vi "SciScan RESONANT.vi"() -> ()   [LabVIEW 2017]
doc: "SciScan 1.1f2 160418"
uses:
  Custom Controls/Ch selector.ctl
  Custom Controls/MAIN Image panel reso tab Control type def.ctl
  Custom Controls/scan mode main settings tab.ctl
  Custom Controls/advanced settings inner tab CTL.ctl
  Custom Controls/Laser power 1 dial.ctl
  Custom Controls/Histogram tab reso.ctl
  Custom Controls/file format type def.ctl
  Custom Controls/display palette control.ctl
  Custom Controls/PositionSaveMod.ctl
  Custom Controls/pixel resolution resonant enum.ctl
  Custom Controls/experiment type.ctl
  HFG/Custom Controls and Typedefs/HFG Commands.ctl
  CommonResource VIs/Timing/Timer Commands.ctl
  HFG/SubVIs/Broken Chain FGV Command.ctl
  Plugins/Macro Module/Macro Rule/subVIs/MacroRules_FGV_Commands.ctl
  Plugins/Macro Module/Macro Rule/subVIs/MacroErrorsFGV_Commands.ctl
  <vilib>/event_ctls.llb/lveventtype.ctl
  INI/settingsIO/Settings IO_Commands.ctl
  Plugins/Macro Module/MacroGUI Module/Custom Controls and Typedefs/GFG Variable for IO.ctl
  <vilib>/Utility/miscctls.llb/LVMinMaxIncTypeDef.ctl
  <vilib>/Utility/miscctls.llb/LVOutOfRangeActionTypeDef.ctl
  <vilib>/DAQmx/write.llb/DAQmx Write (Analog DBL 1Chan 1Samp).vi
  GFG/GFGfpRefGet.vi
  <vilib>/DAQmx/miscellaneous.llb/DAQmx Fill In Error Info.vi
  GFG/GFGnumericGet.vi
  GFG/GFGpathGet.vi
  GFG/GFGstringGet.vi
  GFG/GFG library.lvlib
panel:
  in  "MAIN UI responsive? (F)":bool
  in  "shutterlock":bool caption="LOCK"
  in  "custom step z":bool
  in  "custom step xy":bool
  in  "no of grid lines":dbl(slide) min=0.0 step=1.0 scale=0.0..20.0
  out "grid size":string caption="GRID"
  in  "save prot":bool
  in  "piezo.active":bool
  in  "lasersync.enable":bool
  in  "resonant.correction.enable":bool
  in  "PositionSaveButton":T1
  in  "reset zoom":bool
  in  "bool.stage.speed":bool=TRUE
  in  "x.voltage":dbl=0.9999999999999999 min=0.0 max=5.5 step=0.1
  in  "y.voltage":dbl=1.0 min=0.0 max=5.5 step=0.1
  in  "y.volt.offset":dbl=-0.2 step=0.1
  in  "x.volt.offset":dbl=-0.2 step=0.1
  in  "shutter":bool
  in  "x.pixels":i32=256 min=2 max=2048 step=2
  in  "clear prot":bool
  in  "timestamp.prot":bool
  in  "protocol.notes":string caption="notebook"
  in  "Open All\nSettings":bool=TRUE
  in  "step.size.z":u16(ring)=1 items=["    1"=1, "    2"=2, "    5"=5, "  10"=10, "  20"=20, "100"=100]
  in  "Stage Stop":bool
  out "frame count":dbl(slide) scale=0.0..100.0
  in  "scan mode main settings":T2
  in  "pixel resolution":T3=enum."512 x 512"
  in  "autocorrect.startdelay":bool
  in  "x.correction":dbl(slide)=-27.0 min=-200.0 max=200.0 step=1.0 scale=-200.0..200.0 scale format="%#_3g"
  in  "ZOOM":dbl(slide)=1.0 min=1.0 max=20.1 step=0.125 scale=1.0..20.0
  in  "Start.Delay":dbl(slide)=1.0 min=1.0 max=2500.0 step=1.0 scale=1.0..2500.0 scale format="%#_3f"
  in  "no. of frames to acquire":i32=10000 min=4 max=1000000 step=4
  out "x.fov":dbl caption="Field of view    x" format="%#_3p"
  out "y.fov":dbl caption="y" format="%#_3p"
  out "frames.p.sec":dbl caption="frames/s" format="%#.2g"
  in  "invert.ch.4":bool
  in  "save.ch.4":bool caption="ch 4"
  in  "invert.ch.3":bool
  in  "save.ch.3":bool caption="ch 3"
  in  "invert.ch.2":bool
  in  "save.ch.2":bool caption="ch 2"
  in  "invert.ch.1":bool
  in  "save.ch.1":bool caption="ch 1"
  in  "experiment name":string
  in  "root.path":path=path "d:/"
  in  "file format":T4
  in  "experiment type":T5="XYT"
  in  "Objective":u16(ring) items=["Olympus 10x", "Olympus 60x", "Nikon 16x", "Olympus 25x"]
  out "stack.duration":i32=10 caption="stack.duration (sec)" min=0 max=2147483646 step=2
  in  "add":bool
  in  "clear all":bool
  in  "clear last":bool
  in  "move to z.stack.\nstart plane":bool
  in  "start z.stack":bool
  in  "frames.per.plane":i32=10000 min=4 max=1000000 step=4
  in  "z.spacing":dbl=1.0 caption="z.spacing (um)" min=0.1 step=0.1
  out "no of planes":i32=10 min=0 max=2147483646 step=2
  in  "piezo.mode":bool
  out "volume rate (in Hz)":dbl=1.0 min=0.0 max=5.5 step=0.1 format="%#.2g"
  in  "frames.per.z.cycle":dbl=4.0 min=4.0 step=2.0
  in  "no.of.cycles.to.scan":dbl=2.0 caption="no.of.volumes" min=1.0 step=1.0
  in  "piezo.offset.compensation.seconds":dbl caption="no.of.volumes"
  in  "Z UP":bool
  in  "Z DOWN":bool
  out "String 7":string
  in  "step.size.xy":u16(ring)=1 items=["   1"=1, "   2"=2, "   5"=5, "  10"=10, "  20"=20, "  50"=50, "100"=100]
  in  "Y UP":bool
  in  "X LEFT":bool
  in  "Y DOWN":bool
  in  "X RIGHT":bool
  out "String 6":string
  in  "setY":dbl caption="Z-Stepper" format="%#.1f"
  in  "setX":dbl caption="Z-Stepper" format="%#.1f"
  in  "setZ":dbl caption="set" format="%#.1f"
  out "String 4":string
  out "posZ":dbl caption="actual" format="%#.1f"
  out "posX":dbl caption="Z-Stepper" format="%#.1f"
  out "posY":dbl caption="Z-Stepper" format="%#.1f"
  out "String 3":string
  in  "QUIT":bool
  in  "Record":bool
  in  "FOCUS":bool
  in  "MAIN Image panels reso":T6
  out "Channel 1 large":T7(plugin-control)
  out "Channel 2 large":T7(plugin-control)
  out "Channel 3 large":T7(plugin-control)
  out "Channel 4 large":T7(plugin-control)
  out "Channel 5 large":T7(plugin-control)
  out "Channel 1 small":T7(plugin-control)
  out "Channel 2 small":T7(plugin-control)
  out "Channel 4 small":T7(plugin-control)
  out "Channel 3 small":T7(plugin-control)
  in  "Blue Channel (Overlay)":T8 caption="B"
  in  "Green Channel (Overlay)":T8=enum."Ch 1" caption="G"
  in  "Red Channel (Overlay)":T8=enum."Ch 2" caption="R"
  out "RGB overlay":T7(plugin-control)
  out "ROI chart":sgl[][](graph)=[[54.570076, 54.556858]]
  in  "ROI channel":T8=enum."Ch 1" caption="Channel"
  out "ROI Image display":T7(plugin-control)
  in  "confirm line":bool
  in  "channel arb line scan":T8 caption="Channel"
  out "arb line scan display":T7(plugin-control)
  in  "Cancel":bool
  in  "hist/ref slider tab":enum32{" "}(tab)
  in  "display every n-th frame":i8=4 min=2 step=1
  in  "PIN Button hist/ref slider tab":bool=TRUE
  in  "Histograms tab reso":T9
  in  "auto scale\n      CH 1":bool=TRUE caption="auto scale 2"
  in  "Min Max Channel 1":cluster{dbl, dbl}(slide)={0.0, 65535.0} scale=0.0..65535.0 scale format="%#_5g"
  out "Histogram 1":T10(graph)
  out "String 12":string
  in  "auto scale\n      CH 4":bool=TRUE caption="auto scale 2"
  in  "Min Max Channel 4":cluster{dbl, dbl}(slide)={0.0, 65535.0} scale=0.0..65535.0 scale format="%#_5g"
  out "Histogram 4":T10(graph)
  out "String 15":string
  in  "auto scale\n      CH 5":bool=TRUE caption="auto scale 2"
  in  "Min Max Channel 5":cluster{dbl, dbl}(slide) scale=-100.0..2047.0 scale format="%#_4g"
  out "Histogram 5":T10(graph)
  out "String 16":string
  in  "auto scale\n      CH 3":bool=TRUE caption="auto scale 2"
  in  "Min Max Channel 3":cluster{dbl, dbl}(slide)={0.0, 65535.0} scale=0.0..65535.0 scale format="%#.1f"
  out "Histogram 3":T10(graph)
  out "String 14":string
  in  "auto scale\n      CH 2":bool=TRUE caption="auto scale 2"
  in  "Min Max Channel 2":cluster{dbl, dbl}(slide)={0.0, 65535.0} scale=0.0..65535.0 scale format="%#.0f"
  out "Histogram 2":T10(graph)
  out "String 13":string
  in  "avg type":u16(ring) items=["none", "group avg", "moving avg"]
  in  "avg of":i8=10 min=2 step=1
  in  "display palette":T11
  in  "large histogram":bool caption="Pop-Out"
  in  "laser power slider tab":enum32{""}(tab)
  in  "enable set power max":bool
  in  "set power max":bool
  in  "Laser Power":T12 min=0.0 max=100.0 step=0.5 scale=0.0..100.0 scale format="%3d"
  in  "PIN Button laser power slider tab":bool=TRUE
  in  "blanking\npercentage":i32=90 min=0 max=90 step=1
  in  "PMT slider tab":enum32{""}(tab)
  in  "PMT 2":u16(slide) max=1000 scale=0.0..1000.0
  in  "PMT 1":u16(slide) max=1250 scale=0.0..1000.0
  out "String 5":string
  in  "PMT 4":u16(slide) max=1000 scale=0.0..1000.0
  in  "PMT 3":u16(slide) max=1250 scale=0.0..1000.0
  out "String 18":string
  in  "PIN Button PMT slider tab":bool=TRUE
  in  "advanced settings slider tab":enum32{""}(tab)
  in  "advanced settings inner tab":T13
  in  "y.pixel.sz":dbl=1e-05 min=1e-09 max=1e-05 step=1e-07 format="%#_3p"
  in  "x.pixel.sz":dbl=1e-05 min=1e-09 max=1e-05 step=1e-07 format="%#_3p"
  in  "y.pixels":i32=512 caption="Y Resolution" min=60 max=2048 step=2
  in  "nomin.x.pixels":i32=512 caption="X resolution" min=2 max=2048 step=2
  in  "voltage.for\nmin.field.of.view\nresonant":dbl=5.0 caption="voltage.for min.field.of.view resonant"
  in  "max.field.of.view\nresonant":dbl=300.0 caption="max.field.of.view resonant" format="%#_6p"
  in  "voltage.for\nmax.field.of.view\nresonant":dbl=5.0 caption="voltage.for max.field.of.view resonant"
  in  "max.field.of.view":dbl=300.0 format="%#_6p"
  in  "voltage.for\nmax.field.of.view":dbl=5.0
  in  "external.start.trigger.enable":bool=TRUE caption="WAIT FOR TRIGGER"
  in  "abs/rel z pos":enum32{"abs", "rel"}(tab)
  in  "pos  pockels cell PMT Data":dbl[][](array[numeric]) caption="Data" format="%0.1f"
  in  "RELATIVE pos  pockels cell PMT Data":dbl[][](array[numeric]) caption="Data" format="%0.1f"
  in  "PIN Button advanced settings slider tab":bool=TRUE
  in  "XYZ stage settings slider tab":enum32{" "}(tab)
  in  "LP enable":bool
  out "String 20":string
  in  "set stage speed":bool
  in  "enable virtual XYZ":bool
  out "String 19":string
  in  "set X to zero":bool
  in  "set Y to zero":bool
  in  "set all to zero":bool
  in  "set Z to zero":bool
  out "String 9":string
  in  "reverse x":bool
  in  "reverse y":bool
  in  "reverse z":bool
  out "String 8":string
  in  "PIN Button XYZ stage settings slider tab":bool=TRUE
  in  "SCIENTIFICA Button":bool
  # "to zoom out press and hold Shift"
  # "OFF"
  # "2x2"
  # "4x4"
  # "6x6"
  # "8x8"
  # "10x10"
  # "12x12"
  # "14x14"
  # "16x16"
  # "18x18"
  # "20x20"
  # "abs pos."
  # "x"
  # "y"
  # "z"
  # "x"
  # "y"
  # "z"
  # "rel pos."
  # "auto"
  # "adj."
  # "Active channels"
  # "Invert channels"
  # "Z Stack parameters"
  # "Z Stack plane management"
  # "zig-zag (leaf scan)"
  # "sawtooth"
  # "Typically, the response lag of piezo positioning is in the millisecond range. Use negative values to compensate for this lag.  Example: -0.015 seconds"
  # "1"
  # "2"
  # "3"
  # "4"
  # "Press and hold Ctrl to add multiple ROIs"
  # "Y scanner (Galvo)"
  # "Adjust aspect ratio between X and Y here"
  # "X scanner (Reso)"
  # "This checkbox is only for starting the image acquisition using a TTL rising edge trigger from an external device. Connect to DI1 (NI 5751) or DIO 0.1 (NI 5734).\n\nIf you want to send a trigger to an external device, use DO0-2 (NI 5751) or DIO 1.0-1.2 (NI 5734), but leave the  checkbox above unticked."
  # "X"
  # "Y"
  # "Z"
  # "LASER1"
  # "LASER2"
  # "X"
  # "Y"
  # "Z"
  # "LASER1"
  # "LASER2"
  # "reverse \ndirection"
  # "Zero\nrel. pos."
  # "z"
  # "x"
  # "y"
  # "LP enable"
  # "virtual XYZ"
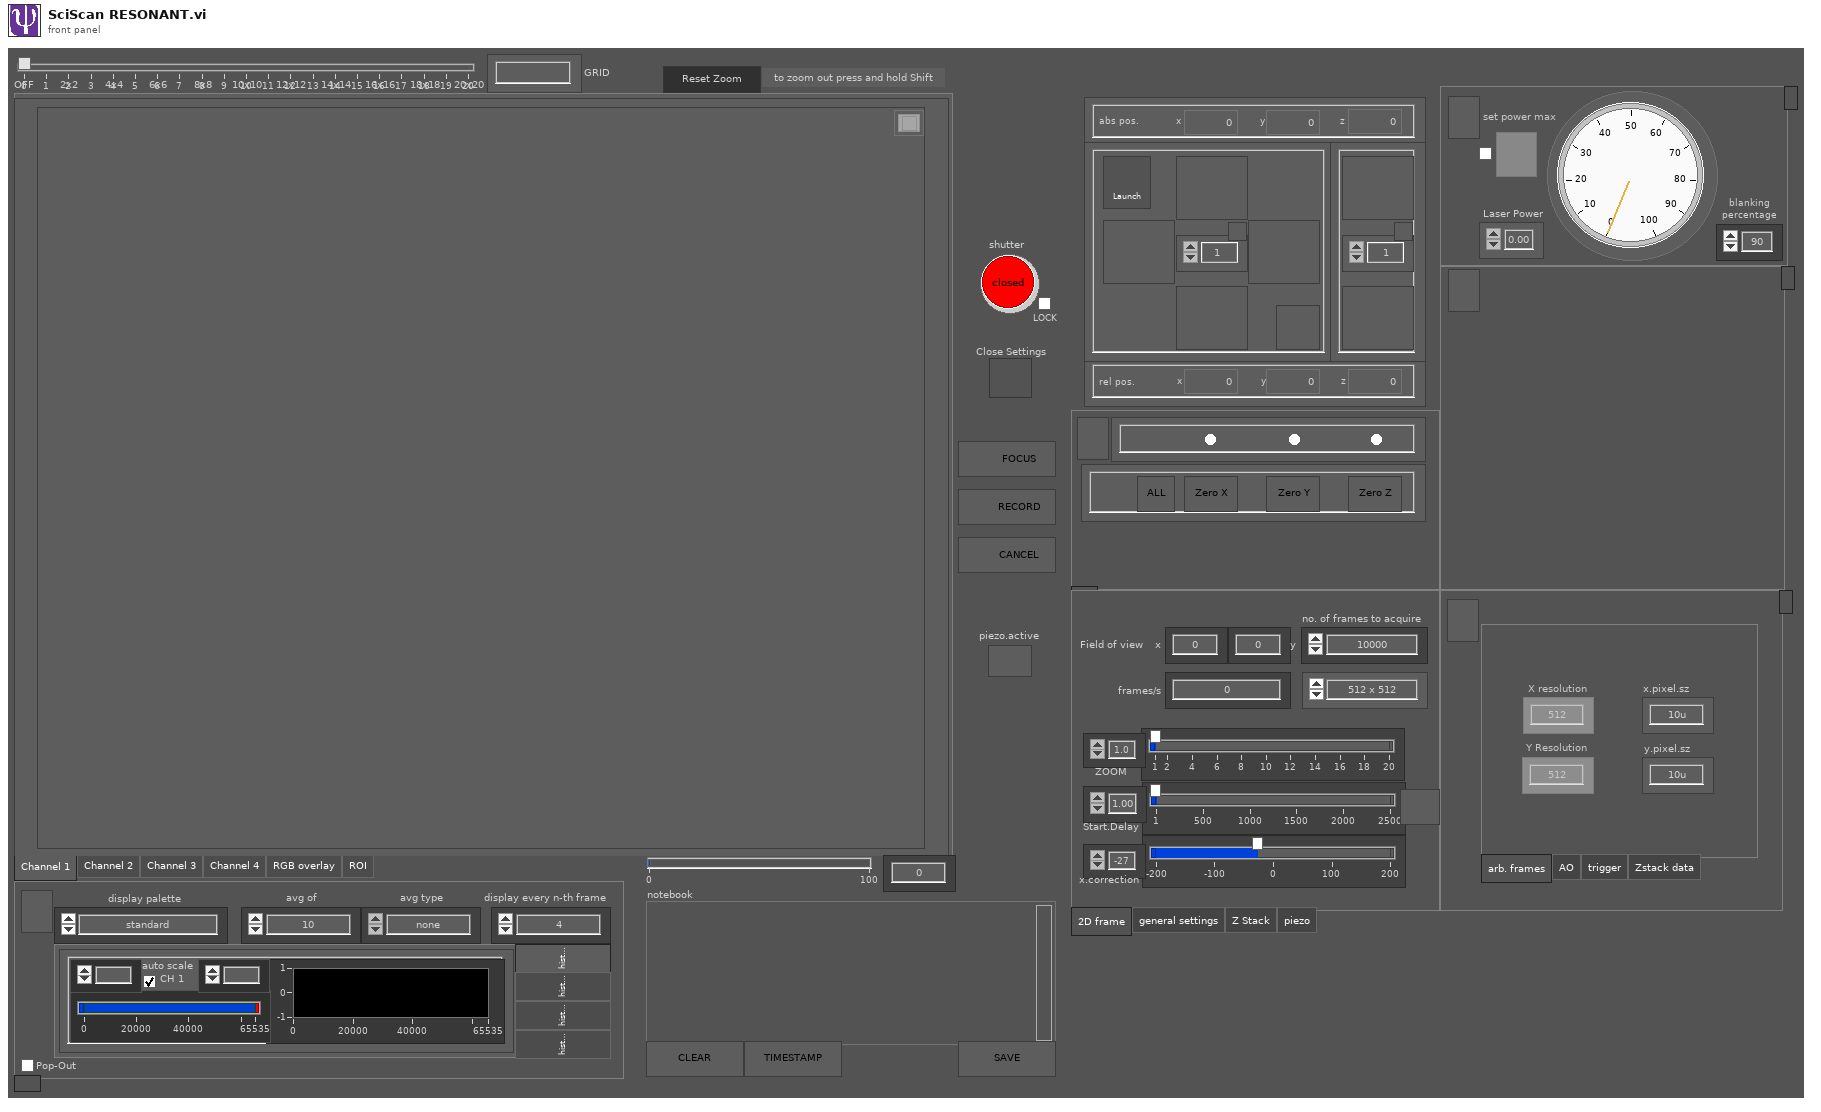
[diagram p1: front panel]
types:
  T1 = typedef "PositionSaveMod.ctl" = bool
  T2 = typedef "scan mode main settings tab.ctl" = enum32{"2D frame", "2D line scan", "general settings", "Z Stack", "piezo"}
  T3 = typedef "pixel resolution resonant enum.ctl" = enum16{"512 x  64", "512 x 128", "512 x 256", "512 x 512", "512 x arbitrary", "1024 x 512", "1024 x 1024", " 1024 x arbitrary", " 1536 x  512", " 1536 x arbitrary"}
  T4 = typedef "file format type def.ctl" = enum16{"16bit raw", "32bit raw", "16bit multi-tiff (interleave)", "16bit multi-tiff (separate)", "16bit multi-tiff (stacked)", "32bit multi-tiff (interleave)", "32bit multi-tiff (separate)", "32bit multi-tiff (stacked)", "16bit tiff series (interleave)", "16bit tiff series (separate)", "16bit tiff series (stacked)", "32bit tiff series (interleave)", "32bit tiff series (separate)", "32bit tiff series (stacked)"}
  T5 = typedef "experiment type.ctl" = string
  T6 = typedef "MAIN Image panel reso tab Control type def.ctl" = enum32{"Channel 1", "Channel 2", "Channel 3", "Channel 4", "Channel 5", "all channels", "RGB overlay", "ROI", "arbitrary line scan"}
  T7 = typedef "IMAQ Image.ctl" = refnum<image>
  T8 = typedef "Ch selector.ctl" = enum16{"none", "Ch 1", "Ch 2", "Ch 3", "Ch 4"}
  T9 = typedef "Histogram tab reso.ctl" = enum32{"hist Ch 1", "hist Ch 4", "hist Ch 5", "hist Ch 3", "hist Ch 2"}
  T10 = cluster{"Starting Value":sgl, "Incremental Value":sgl, "Histogram":u32[]}
  T11 = typedef "display palette control.ctl" = enum16{"standard", "high clipping red", "low clipping blue", "high and low clipping", "high / low (full range)"}
  T12 = typedef "Laser power 1 dial.ctl" = dbl
  T13 = typedef "advanced settings inner tab CTL.ctl" = enum32{"arb. frames", "AO", "AI", "channels", "trigger", "Zstack data"}
  T14 = enum16{"Get Settings Table ", "Read Settings File", "Get Specified Settings"}
  T15 = typedef "MacroErrorsFGV_Commands.ctl" = enum16{"Initialize", "Get Error Array", "Set Error Array"}
  T16 = typedef "MacroRules_FGV_Commands.ctl" = enum16{"Read File", "Get All", "Get Param and Flags"}
  T17 = typedef "Broken Chain FGV Command.ctl" = enum16{"Initialize", "Update VI status", "Get All VI status"}
  T18 = typedef "Timer Commands.ctl" = enum16{"Clear All", "Start", "Pause", "Check Time"}
  T19 = typedef "HFG Commands.ctl" = enum16{"Set", "Get", "Initialize"}
  T20 = enum8{"Enabled", "Disabled", "Disabled and Grayed Out"}
  T21 = typedef "Image Type" = u32
  T22 = cluster{refnum<vi>, refnum<vi>, refnum<vi>, refnum<vi>, refnum<vi>, refnum<vi>, refnum<vi>, refnum<vi>, refnum<vi>, refnum<vi>, refnum<vi>, refnum<vi>}
  T23 = cluster{"New Image":T7, "New Image":T7, "New Image":T7, "New Image":T7, "New Image":T7, "New Image":T7, "New Image":T7, "New Image":T7, "New Image":T7, "New Image":T7, "New Image":T7, "New Image":T7}
  T24 = typedef "LVMinMaxIncTypeDef.ctl" = cluster{"Minimum":dbl, "Maximum":dbl, "Increment":dbl}
  T25 = typedef "LVOutOfRangeActionTypeDef.ctl" = cluster{"Out of Range Action Minimum":u8, "Out of Range Action Maximum":u8, "Out of Range Action Increment":u8}
  T26 = typedef "lveventtype.ctl" = enum32{"Null", "Timeout", "Annotation Menu Selection", "Annotation Menu Selection?", "App Instance Close", "App Instance Close?", "Autoscale Range Change", "Bookmark Info Change", "Cell Edit", "Cell Edit?", "Cursor Grab", "Cursor Grab?", "Cursor Menu Selection", "Cursor Menu Selection?", "Cursor Move", "Cursor Release", "Data Change", "Direction Change", "Display State Change", "Drag Ended", "Drag Enter", "Drag Leave", "Drag Over", "Drag Source Update", "Drag Starting", "Drag Starting?", "Drop", "Exec State Change", "Key Down", "Key Down?", "Key Repeat", "Key Repeat?", "Key Up", "Listbox Double Click", "Menu Activation?", "Menu Selection (App)", "Menu Selection? (App)", "Menu Selection (User)", "Mouse Down", "Mouse Down?", "Mouse Enter", "Mouse Leave", "Mouse Move", "Mouse Up", "Mouse Wheel", "NI Security User Change (App)", "Pane Size", "Panel Close", "Panel Close?", "Panel Resize", "Plot Attribute Change", "Scale Range Change", "Shortcut Menu Activation?", "Shortcut Menu Selection (App)", "Shortcut Menu Selection? (App)", "Shortcut Menu Selection (User)", "Tree Double Click", "Tree Drag", "Tree Drag?", "Tree Drop", "Tree Drop?", "Tree Item Close", "Tree Item Close?", "Tree Item Open", "Tree Item Open?", "User Event", "Value Change"}
  T27 = enum32{"Invalid", "Standard", "Closed", "Hidden", "Minimized", "Maximized"}
  T28 = enum32{"Invalid", "Default", "Floating", "Floating/Auto-Hide", "Modal"}
  T29 = typedef "Settings IO_Commands.ctl" = enum16{"Write HW Settings", "Write Config Settings", "Read HW Settings", "Read Config Settings", "Write Line-Scan Settings", "Write Frame-Scan Settings", "Write Z-Stack Settings", "Read Line-Scan Settings", "Read Frame-Scan Settings", "Read Z-Stack Settings", "Read Fast-Z Settings", "Write Fast-Z Settings"}
  T30 = typedef "GFG Variable for IO.ctl" = cluster{"Variable Name":string, "Value (Variant)":variant, "data type":string}
  T31 = cluster{"WaveformChartRef":refnum<vi>, "DigitalRef":refnum<vi>, "ArrayRef":refnum<vi>, "TabControlRef":refnum<vi>, "EnumRef":refnum<vi>, "RingRef":refnum<vi>, "BooleanRef":refnum<vi>, "KnobRef":refnum<vi>, "SlideRef":refnum<vi>, "PathRef":refnum<vi>, "StringRef":refnum<vi>, "ComboBox":refnum<vi>, "WaveformGraphRef":refnum<vi>}
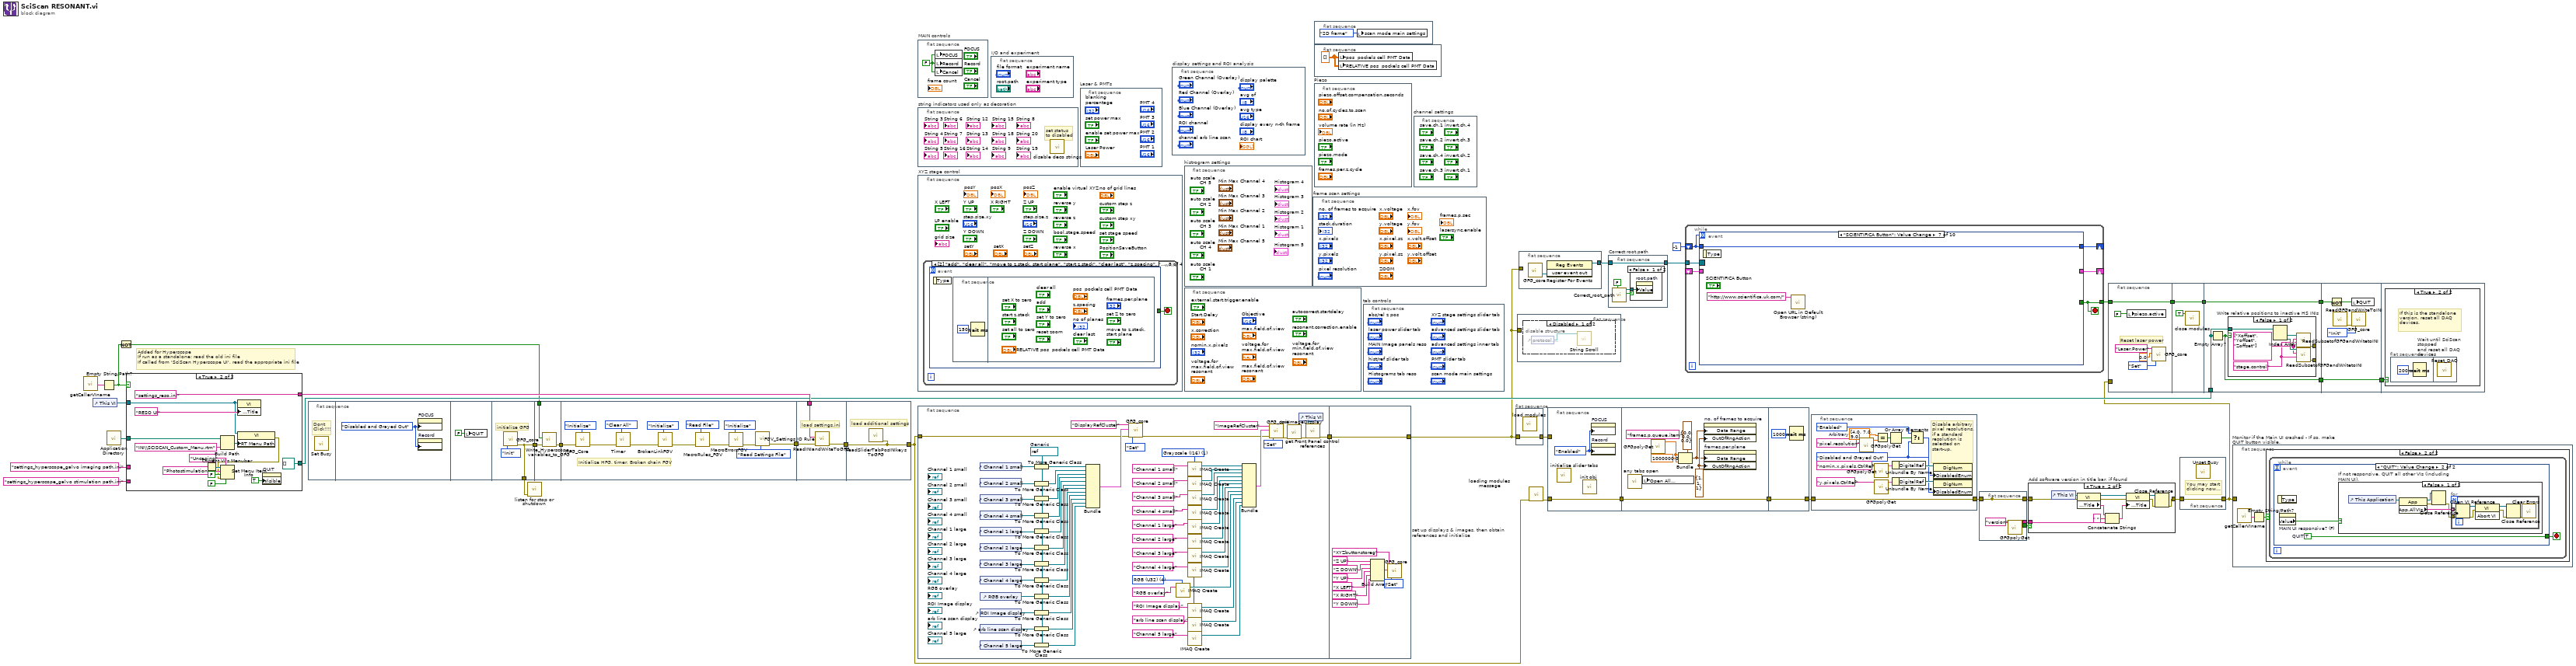
[diagram p0: block diagram]
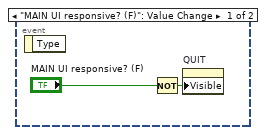
[diagram p3: hidden frame]
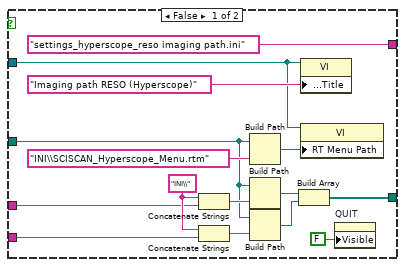
[diagram p6: hidden frame]
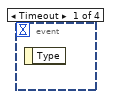
[diagram p9: hidden frame]
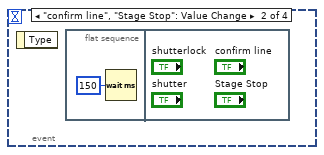
[diagram p10: hidden frame]
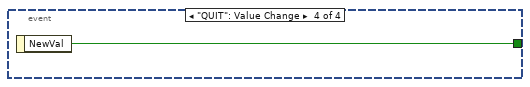
[diagram p11: hidden frame]
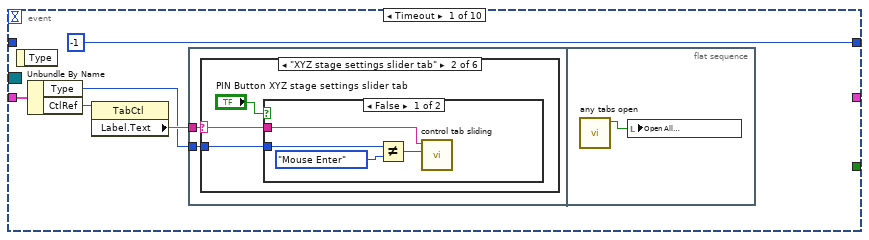
[diagram p14: hidden frame]
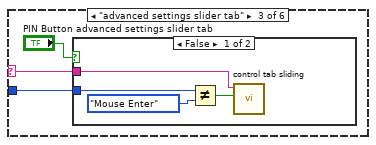
[diagram p17: hidden frame]
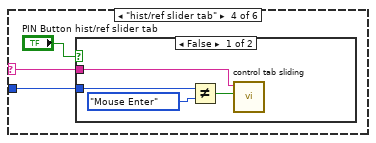
[diagram p19: hidden frame]
diagram:
  # "Added for Hyperscope\nIf run as a standalone; read the old ini file\nIf called from 'SciScan Hyperscope UI', read the appropriate ini file"
  n1 = call "getCallerVIname.vi"() -> ("VI name"=w25:string)  [unwired: 19 in]
  n2 = control-ref of="This VI"() -> (w3:refnum<vi>)
  n3 = Empty String/Path?(string/path=w25) -> (empty?=w2:bool)
  n4 = call <vilib>:"Application Directory.vi"() -> ("Application Directory"=w23:path)
  n5 = Not(x=w2) -> (.not. x?=w1:bool)
  n6 = case shown="True" w2 {
    tunnel: ["settings_hyperscope_reso imaging path.ini" ("name or relative path") "settings_reso.ini" ("name or relative path")] -> w24
    tunnel: w3 -> [w48 w61]
    tunnel: w23 -> [w40 w62]
    tunnel: "settings_hyperscope_galvo imaging path.ini" ("name or relative path") -> [w42 _]
    tunnel: "settings_hyperscope_galvo stimulation path.ini" ("name or relative path") -> [w41 _]
    tunnel: [w39 path[] []] -> w17
    frame False {
      w44 = "INI\\" ("name or relative path")
      n7 = Concatenate Strings(w44, w42) -> (w47:string)
      n8 = Concatenate Strings(w44, w41) -> (w46:string)
      n9 = Build Path(base path=w40, name or relative path="INI\\SCISCAN_Hyperscope_Menu.rtm") -> (appended path=w49:path)
      n10 = Build Path(base path=w40, name or relative path=w47) -> (appended path=w45:path)
      n11 = Build Path(base path=w40, name or relative path=w46) -> (appended path=w43:path)
      n12 = Build Array(w45, w43) -> (w39:path[])
      n13 = property class="VI"(reference=w48, "Front Panel.Title"="Imaging path RESO (Hyperscope)" ("Front Panel Window:Title")) -> ()  [unwired: 1 in, 2 out]
      n14 = property class="VI"(reference=w48, "RT Menu Path"=w49) -> ()  [unwired: 1 in, 2 out]
      n15 = property on="QUIT" class="Bool (strict)"("Visible"=FALSE) -> ()  [unwired: 2 in, 2 out]
    }
    frame True {
      n16 = Current VI's Menubar() -> (w54:refnum<k9>)
      n17 = Build Path(base path=w62, name or relative path="INI\\SCISCAN_Custom_Menu.rtm") -> (appended path=w64:path)
      n18 = property class="VI"(reference=w61, "Front Panel.Title"="RESO UI" ("Front Panel Window:Title")) -> ()  [unwired: 1 in, 2 out]
      n19 = property class="VI"(reference=w61, "RT Menu Path"=w64) -> (error out=w53:errorcluster)  [unwired: 1 in, 1 out]
      n20 = Set Menu Item Info(6:FALSE ("checked"), 7:"Uncaging" ("item tag"), 8:w53, 9:FALSE ("enabled"), 10:"Photostimulation" ("name or relative path"), 11:w54) -> ()  [unwired: 1 in, 2 out]
      n21 = property on="QUIT" class="Bool (strict)"("Visible"=TRUE) -> ()  [unwired: 2 in, 2 out]
    }
  }
  n22 = flat-sequence {
    tunnel: [w69] -> w16
    tunnel: [w69] -> w28
    tunnel: w16 -> [w73]
    tunnel: [w72] -> w15
    tunnel: w1 -> [w71]
    tunnel: w15 -> [w77]
    tunnel: [w74] -> w31
    tunnel: w31 -> [w89]
    tunnel: [w88] -> w35
    tunnel: w24 -> [w87]
    tunnel: [w90] -> w5
    tunnel: w35 -> [w90]
    frame #0 {
      # "Dont\nClick!!!!"
      n23 = call <vilib>:"Set Busy.vi"() -> ()  [unwired: 10 in, 2 out]
    }
    frame #1 {
      w67 = T20."Disabled and Grayed Out" ("Disabled")
      n24 = property on="FOCUS" class="Bool (strict)"("DisabledEnum"=w67) -> ()  [unwired: 2 in, 2 out]
      n25 = property on="Record" class="Bool (strict)"("DisabledEnum"=w67) -> ()  [unwired: 2 in, 2 out]
    }
    frame #2 {
      n26 = local write "QUIT"(FALSE ("QUIT")) -> ()
    }
    frame #3 {
      # "initialize GFG"
      n27 = call "GFG_core.vi"("Action"=enum16{"Init", "Set", "Get"}."Init") -> ("error out"=w69:errorcluster)  [unwired: 12 in, 6 out]
    }
    frame #4 {
      n28 = call "Write_Hyperscope_variables_to_GFG.vi"("error in (no error)"=w73, "HyperScope Imaging Path Reso? (F)"=w71) -> ("error out"=w72:errorcluster)  [unwired: 9 in]
    }
    frame #5 {
      # "Initialize HFG, timer, Broken chain FGV"
      n29 = call "HFG_Core.vi"("HFG Commands"=HFG_Commands."Initialize", "Error In"=w77) -> ("Error Out"=w84:errorcluster)  [unwired: 6 in, 3 out]
      n30 = call "Timer.vi"("Timer Command"=Timer_Commands."Clear All", "Error In"=w84) -> ("Error Out"=w82:errorcluster)  [unwired: 4 in, 5 out]
      n31 = call "BrokenLinkFGV.vi"("Broken Chain FGV Action"=Broken_Chain_FGV_Command."Initialize", "Error In"=w82) -> ("Error Out"=w80:errorcluster)  [unwired: 7 in, 2 out]
      n32 = call "MacroRules_FGV.vi"("MacroRules_FGV_Commands"=MacroRules_FGV_Commands."Read File", "Error In"=w80) -> ("Error Out"=w79:errorcluster)  [unwired: 5 in, 4 out]
      n33 = call "MacroErrorsFGV.vi"("MacroErrorsFGV_Commands"=MacroErrorsFGV_Commands."Initialize", "Error In"=w79) -> ("Error Out"=w75:errorcluster)  [unwired: 8 in, 1 out]
      n34 = call "FGV_Settings IO Rule.vi"("Command_Settings IO Rule"=T14."Read Settings File", "Error In"=w75) -> ("Error Out"=w74:errorcluster)  [unwired: 7 in, 2 out]
    }
    frame #6 {
      # "load settings.ini"
      n35 = call "ReadINIandWriteToGFG.vi"("error in (no error)"=w89, "name or relative path"=w87) -> ("error out"=w88:errorcluster)  [unwired: 9 in]
    }
    frame #7 {
      # "load additional settings"
      n36 = call "ReadSliderTabPosINIkeysToGFG.vi"("error in (no error)"=w90) -> ()  [unwired: 11 in]
    }
  }
  n37 = call "listen for stop or shutdown.vi"("error in (no error)"=w28) -> ()  [unwired: 9 in, 2 out]
  n38 = flat-sequence "MAIN controls" {
    frame #0 {
      w91 = FALSE ("FOCUS")
      n39 = local write "FOCUS"(w91) -> ()
      n40 = local write "Record"(w91) -> ()
      n41 = local write "Cancel"(w91) -> ()
    }
  }
  n42 = flat-sequence "string indicators used only as decoration" {
    frame #0 {
      # "set status\nto disabled"
      n43 = call "disable deco strings.vi"() -> ()  [unwired: 11 in, 1 out]
    }
  }
  n44 = flat-sequence "XYZ stage control" {
    frame #0 {
      n45 = while {
        stop <- w92 stop-if-true
        n46 = event shown="[2] \"add\", \"clear all\", \"move to z.stack. start plane\", \"start z.stack\", \"clear last\", \"z.spacing\", \"frames.per.plane\", \"no of planes\", \"set X to zero\", \"set Y to zero\", \"set all to zero\", \"set Z to zero\", \"reset zoom\", \"autocorrect.startdelay\": Value Change" {
          selector: _ -> [_ _ _ _]
          dyn-events: _ -> [_ _ _ _]
          timeout: _ -> [_ _ _ _]
          tunnel: [_ _ _ w95] -> w92
          event Timeout {
            n47 = event-data() -> ()  [unwired: 1 in, 1 out]
          }
          event "confirm line", "Stage Stop": Value Change {
            n48 = event-data() -> ()  [unwired: 1 in, 1 out]
            n49 = flat-sequence {
              frame #0 {
                n50 = Wait (ms)(milliseconds to wait=u32 150) -> ()  [unwired: 1 out]
              }
              frame #1 {
              }
            }
          }
          event "add", "clear all", "move to z.stack.\nstart plane", "start z.stack", "clear last", "z.spacing", "frames.per.plane", "no of planes", "set X to zero", "set Y to zero", "set all to zero", "set Z to zero", "reset zoom", "autocorrect.startdelay": Value Change {
            n51 = event-data() -> ()  [unwired: 1 in, 1 out]
            n52 = flat-sequence {
              frame #0 {
                n53 = Wait (ms)(milliseconds to wait=u32 150) -> ()  [unwired: 1 out]
              }
              frame #1 {
              }
            }
          }
          event "QUIT": Value Change {
            n54 = event-data() -> ("NewVal"=w95:bool)  [unwired: 1 in]
          }
        }
      }
    }
  }
  n55 = flat-sequence "set up displays & images, then obtain references and initialize" {
    tunnel: w5 -> [w114]
    tunnel: [w115] -> w33
    tunnel: [w168] -> w11
    tunnel: w33 -> [w168]
    frame #0 {
      w102 = T21 4 items=["Grayscale (U8)", "Grayscale (I16)", "Grayscale (SGL)", "Complex (CSG)", "RGB (U32)", "HSL (U32)", "RGB (U64)", "Grayscale (U16)"] ("Image Type")
      w97 = T21 1 items=["Grayscale (U8)", "Grayscale (I16)", "Grayscale (SGL)", "Complex (CSG)", "RGB (U32)", "HSL (U32)", "RGB (U64)", "Grayscale (U16)"] ("Image Type")
      w100 = refnum<vi> refnum  # Generic
      n56 = control-ref of="Channel 1 small"() -> (w113:refnum<vi>)
      n57 = control-ref of="Channel 2 small"() -> (w112:refnum<vi>)
      n58 = control-ref of="Channel 3 small"() -> (w111:refnum<vi>)
      n59 = control-ref of="Channel 4 small"() -> (w110:refnum<vi>)
      n60 = control-ref of="Channel 1 large"() -> (w109:refnum<vi>)
      n61 = control-ref of="Channel 2 large"() -> (w108:refnum<vi>)
      n62 = control-ref of="Channel 3 large"() -> (w107:refnum<vi>)
      n63 = control-ref of="Channel 4 large"() -> (w106:refnum<vi>)
      n64 = control-ref of="RGB overlay"() -> (w105:refnum<vi>)
      n65 = control-ref of="ROI Image display"() -> (w104:refnum<vi>)
      n66 = control-ref of="arb line scan display"() -> (w103:refnum<vi>)
      n67 = control-ref of="Channel 5 large"() -> (w101:refnum<vi>)
      n68 = To More Generic Class(target class=w100, reference=w113) -> (generic class reference=w155:refnum<vi>)
      n69 = To More Generic Class(target class=w100, reference=w112) -> (generic class reference=w148:refnum<vi>)
      n70 = To More Generic Class(target class=w100, reference=w111) -> (generic class reference=w147:refnum<vi>)
      n71 = To More Generic Class(target class=w100, reference=w110) -> (generic class reference=w146:refnum<vi>)
      n72 = To More Generic Class(target class=w100, reference=w109) -> (generic class reference=w145:refnum<vi>)
      n73 = To More Generic Class(target class=w100, reference=w108) -> (generic class reference=w154:refnum<vi>)
      n74 = To More Generic Class(target class=w100, reference=w107) -> (generic class reference=w153:refnum<vi>)
      n75 = To More Generic Class(target class=w100, reference=w106) -> (generic class reference=w152:refnum<vi>)
      n76 = To More Generic Class(target class=w100, reference=w105) -> (generic class reference=w151:refnum<vi>)
      n77 = To More Generic Class(target class=w100, reference=w104) -> (generic class reference=w150:refnum<vi>)
      n78 = To More Generic Class(target class=w100, reference=w103) -> (generic class reference=w149:refnum<vi>)
      n79 = To More Generic Class(target class=w100, reference=w101) -> (generic class reference=w99:refnum<vi>)
      n80 = Bundle(w155, w148, w147, w146, w145, w154, w153, w152, w151, w150, w149, w99) -> (w158:T22)  [unwired: 1 in]
      n81 = call "GFG_core.vi"("Variable Name in"="DisplayRefCluster", "Variant in"=w158, "error in (no error)"=w114, "Action"=enum16{"Init", "Set", "Get"}."Set") -> ("error out"=w119:errorcluster)  [unwired: 9 in, 6 out]
      n82 = call "IMAQ Create"("Image Name"="RGB overlay", "Image Type"=w102) -> ("New Image"=w139:T7)  [unwired: 3 in, 1 out]
      n83 = call "IMAQ Create"("Image Name"="Channel 1 small", "Image Type"=w97) -> ("New Image"=w131:T7)  [unwired: 3 in, 1 out]
      n84 = call "IMAQ Create"("Image Name"="Channel 2 small", "Image Type"=w97) -> ("New Image"=w132:T7)  [unwired: 3 in, 1 out]
      n85 = call "IMAQ Create"("Image Name"="Channel 3 small", "Image Type"=w97) -> ("New Image"=w133:T7)  [unwired: 3 in, 1 out]
      n86 = call "IMAQ Create"("Image Name"="Channel 4 small", "Image Type"=w97) -> ("New Image"=w134:T7)  [unwired: 3 in, 1 out]
      n87 = call "IMAQ Create"("Image Name"="Channel 1 large", "Image Type"=w97) -> ("New Image"=w135:T7)  [unwired: 3 in, 1 out]
      n88 = call "IMAQ Create"("Image Name"="Channel 2 large", "Image Type"=w97) -> ("New Image"=w136:T7)  [unwired: 3 in, 1 out]
      n89 = call "IMAQ Create"("Image Name"="Channel 3 large", "Image Type"=w97) -> ("New Image"=w137:T7)  [unwired: 3 in, 1 out]
      n90 = call "IMAQ Create"("Image Name"="Channel 4 large", "Image Type"=w97) -> ("New Image"=w138:T7)  [unwired: 3 in, 1 out]
      n91 = call "IMAQ Create"("Image Name"="ROI Image display", "Image Type"=w97) -> ("New Image"=w140:T7)  [unwired: 3 in, 1 out]
      n92 = call "IMAQ Create"("Image Name"="arb line scan display", "Image Type"=w97) -> ("New Image"=w141:T7)  [unwired: 3 in, 1 out]
      n93 = call "IMAQ Create"("Image Name"="Channel 5 large", "Image Type"=w97) -> ("New Image"=w96:T7)  [unwired: 3 in, 1 out]
      n94 = Bundle("New Image"=w131, "New Image"=w132, "New Image"=w133, "New Image"=w134, "New Image"=w135, "New Image"=w136, "New Image"=w137, "New Image"=w138, "New Image"=w139, "New Image"=w140, "New Image"=w141, "New Image"=w96) -> (w143:T23)  [unwired: 1 in]
      n95 = call "GFG_core.vi"("Variable Name in"="ImageRefCluster", "Variant in"=w143, "error in (no error)"=w119, "Action"=enum16{"Init", "Set", "Get"}."Set") -> ("error out"=w118:errorcluster)  [unwired: 9 in, 6 out]
      n96 = call "InitImageDisplay.vi"("error in (no error)"=w118) -> ("error out"=w117:errorcluster)  [unwired: 10 in]
      n97 = control-ref of="This VI"() -> (w116:refnum<vi>)
      n98 = call "get Front Panel control references.vi"("error in (no error)"=w117, "Main VI"=w116) -> ("error out"=w115:errorcluster)  [unwired: 9 in]
    }
    frame #1 {
      n99 = Build Array("Z UP" ("Variable Name in"), "Z DOWN" ("Variable Name in"), "Y UP" ("Variable Name in"), "X LEFT" ("Variable Name in"), "X RIGHT" ("Variable Name in"), "Y DOWN" ("Variable Name in")) -> (w159:string[])
      n100 = call "GFG_core.vi"("Variable Name in"="XYZbuttonstoreg", "Variant in"=w159, "Action"=enum16{"Init", "Set", "Get"}."Set") -> ()  [unwired: 10 in, 7 out]
    }
  }
  n101 = flat-sequence "I/O and experiment" {
    frame #0 {
    }
  }
  n102 = flat-sequence "Laser & PMTs" {
    frame #0 {
    }
  }
  n103 = flat-sequence "display settings and ROI analysis" {
    frame #0 {
    }
  }
  n104 = flat-sequence "histrogram settings" {
    frame #0 {
    }
  }
  n105 = flat-sequence {
    frame #0 {
    }
  }
  n106 = flat-sequence "frame scan settings" {
    frame #0 {
    }
  }
  n107 = flat-sequence "Piezo" {
    frame #0 {
    }
  }
  n108 = flat-sequence {
    frame #0 {
      n109 = local write "scan mode main settings"(scan_mode_main_settings_tab."2D frame" ("scan mode main settings")) -> ()
    }
  }
  n110 = flat-sequence {
    frame #0 {
      w170 = dbl[][] []
      n111 = local write "pos  pockels cell PMT Data"(w170) -> ()
      n112 = local write "RELATIVE pos  pockels cell PMT Data"(w170) -> ()
    }
  }
  n113 = flat-sequence "tab controls" {
    frame #0 {
    }
  }
  n114 = flat-sequence "channel settings" {
    frame #0 {
    }
  }
  n115 = flat-sequence {
    tunnel: w11 -> [w171]
    tunnel: [w171] -> w34
    frame #0 {
      n116 = call "load modules.vi"() -> ()  [unwired: 12 in]
    }
  }
  n117 = flat-sequence {
    tunnel: w11 -> [_]
    frame #0 {
      n118 = disable-structure shown="Disabled" {
        frame Disabled {
          n119 = control-ref of="protocol.notes"() -> (w172:refnum<vi>)
          n120 = call "String Scroll.vi"("fp string refnum in"=w172) -> ()  [unwired: 11 in]
        }
        frame Enabled {
        }
      }
    }
  }
  n121 = flat-sequence {
    tunnel: [w174] -> w27
    tunnel: w11 -> [_]
    frame #0 {
      n122 = call "GFG_core.vi"() -> ("user event out"=w173:refnum<user-event>)  [unwired: 13 in, 6 out]
      n123 = register-events(w173) -> (reference out=w174:refnum<event-registration>)  [unwired: 2 in, 1 out]
    }
  }
  n124 = call "loading modules message.vi"("error in"=w5) -> ("error out"=w32:errorcluster)  [unwired: 10 in]
  n125 = flat-sequence {
    tunnel: w34 -> [_]
    tunnel: w32 -> [w175]
    tunnel: [w175] -> w30
    tunnel: w30 -> [w184]
    tunnel: [w184] -> w22
    tunnel: w22 -> [w186]
    tunnel: [w186] -> w8
    frame #0 {
      w176 = T20."Enabled" ("Disabled")
      n126 = call "initialize slider tabs.vi"() -> ()  [unwired: 12 in]
      n127 = call "init obj.vi"() -> ()  [unwired: 12 in]
      n128 = property on="FOCUS" class="Bool (strict)"("DisabledEnum"=w176) -> ()  [unwired: 2 in, 2 out]
      n129 = property on="Record" class="Bool (strict)"("DisabledEnum"=w176) -> ()  [unwired: 2 in, 2 out]
    }
    frame #1 {
      w179 = T25 {"Out of Range Action Minimum"=1, "Out of Range Action Maximum"=1, "Out of Range Action Increment"=1} ("Response to Value Outside Limits")
      n130 = call "any tabs open.vi"() -> ("any tabs open?"=w177:bool)  [unwired: 11 in]
      n131 = local write "Open All\nSettings"(w177) -> ()
      n132 = call-poly "GFGpolyGet.vi"("Variable Name in"="frames.p.queue.item") -> ("Numeric"=w181:dbl)  [unwired: 8 in, 2 out]
      n133 = Bundle(cluster=T24 {"Minimum"=0.0, "Maximum"=0.0, "Increment"=0.0} ("Data Entry Limits"), "Minimum"=w181, "Maximum"=1000000.0, "Increment"=w181) -> (w178:T24)
      n134 = property on="no. of frames to acquire" class="DigNum (strict)"("Data Range"=w178, "OutOfRngAction"=w179) -> ()  [unwired: 2 in, 2 out]
      n135 = property on="frames.per.plane" class="DigNum (strict)"("Data Range"=w178, "OutOfRngAction"=w179) -> ()  [unwired: 2 in, 2 out]
    }
    frame #2 {
      n136 = Wait (ms)(milliseconds to wait=u32 1000) -> ()  [unwired: 1 out]
    }
  }
  n137 = flat-sequence "Correct root.path" {
    tunnel: w27 -> [w190]
    tunnel: [w190] -> w26
    frame #0 {
      n138 = call "Correct_root_path.vi"("Display warning? (T)"=FALSE) -> ("Path is correct?"=w189:bool, "Resulting path"=w188:path)  [unwired: 8 in, 1 out]
      n139 = case shown="False" w189 {
        tunnel: w188 -> [w191 _]
        frame False {
          n140 = property on="root.path" class="Path"("Value"=w191) -> ()  [unwired: 2 in, 2 out]
        }
        frame True {
        }
      }
    }
  }
  n141 = while {
    tunnel: [w197] -> w37
    shift-right: [w196] -> _
    shift-left: _ -> [w194]
    shift-right: [w195] -> _
    shift-left: -1 -> [w193]
    tunnel: w26 -> [w192]
    stop <- w197 stop-if-true
    n142 = event shown="[6] \"SCIENTIFICA Button\": Value Change" {
      selector: w192 -> [_ _ _ _ _ _ _ _ _ _]
      dyn-events: _ -> [_ _ _ _ _ _ _ _ _ _]
      timeout: w193 -> [_ _ _ _ _ _ _ _ _ _]
      tunnel: [_ w242 _ _ _ "QUIT" _ _ _ _] -> w197
      tunnel: [_ _ _ _ _ _ _ w429 _ _] -> w196
      tunnel: [-1 -1 w248 w276 w386 w408 w425 w432 w444 w486] -> w195
      tunnel: w194 -> [w202 _ _ _ _ _ _ w428 _ _]
      tunnel: w193 -> [_ _ w248 w276 w386 w408 w425 w431 w444 w486]
      event Timeout {
        n143 = event-data() -> ()  [unwired: 1 in, 1 out]
        n144 = Unbundle By Name(w202) -> ("Type"=w199:T26, "CtlRef"=w201:refnum<vi>)
        n145 = property class="TabCtl"(reference=w201) -> ("Label.Text"=w200:string)  [unwired: 1 in, 2 out]
        n146 = flat-sequence {
          tunnel: w200 -> [w204]
          tunnel: w199 -> [w203]
          frame #0 {
            n147 = case shown="\"XYZ stage settings slider tab\"" w204 {
              selector: w204 -> [_ w207 w212 w221 w226 w235]
              tunnel: w203 -> [_ w206 w213 w219 w227 w234]
              frame "False", Default {
              }
              frame "XYZ stage settings slider tab" {
                n148 = case shown="False" "PIN Button XYZ stage settings slider tab" {
                  tunnel: w207 -> [w211 _]
                  tunnel: w206 -> [w210 _]
                  frame False {
                    n149 = Not Equal?(x=w210, y=lveventtype."Mouse Enter" ("Type")) -> (x != y?=w209:bool)
                    n150 = call "control tab sliding.vi"("close(T)/open(F)"=w209, "String"=w211) -> ()  [unwired: 10 in]
                  }
                  frame True {
                  }
                }
              }
              frame "advanced settings slider tab" {
                n151 = case shown="False" "PIN Button advanced settings slider tab" {
                  tunnel: w212 -> [w218 _]
                  tunnel: w213 -> [w217 _]
                  frame False {
                    n152 = Not Equal?(x=w217, y=lveventtype."Mouse Enter" ("Type")) -> (x != y?=w216:bool)
                    n153 = call "control tab sliding.vi"("close(T)/open(F)"=w216, "String"=w218) -> ()  [unwired: 10 in]
                  }
                  frame True {
                  }
                }
              }
              frame "hist/ref slider tab" {
                n154 = case shown="False" "PIN Button hist/ref slider tab" {
                  tunnel: w221 -> [w225 _]
                  tunnel: w219 -> [w224 _]
                  frame False {
                    n155 = Not Equal?(x=w224, y=lveventtype."Mouse Enter" ("Type")) -> (x != y?=w223:bool)
                    n156 = call "control tab sliding.vi"("close(T)/open(F)"=w223, "String"=w225) -> ()  [unwired: 10 in]
                  }
                  frame True {
                  }
                }
              }
              frame "laser power slider tab" {
                n157 = case shown="False" "PIN Button laser power slider tab" {
                  tunnel: w226 -> [w232 _]
                  tunnel: w227 -> [w231 _]
                  frame False {
                    n158 = Not Equal?(x=w231, y=lveventtype."Mouse Enter" ("Type")) -> (x != y?=w230:bool)
                    n159 = call "control tab sliding.vi"("close(T)/open(F)"=w230, "String"=w232) -> ()  [unwired: 10 in]
                  }
                  frame True {
                  }
                }
              }
              frame "PMT slider tab" {
                n160 = case shown="False" "PIN Button PMT slider tab" {
                  tunnel: w235 -> [w239 _]
                  tunnel: w234 -> [w238 _]
                  frame False {
                    n161 = Not Equal?(x=w238, y=lveventtype."Mouse Enter" ("Type")) -> (x != y?=w237:bool)
                    n162 = call "control tab sliding.vi"("close(T)/open(F)"=w237, "String"=w239) -> ()  [unwired: 10 in]
                  }
                  frame True {
                  }
                }
              }
            }
          }
          frame #1 {
            n163 = call "any tabs open.vi"() -> ("any tabs open?"=w240:bool)  [unwired: 11 in]
            n164 = local write "Open All\nSettings"(w240) -> ()
          }
        }
      }
      event User Event {
        n165 = event-data() -> ("Variable Name"=w244:string, "Variant"=w243:variant)  [unwired: 1 in, 1 out]
        n166 = case shown="\"root.path\"" w244 {
          tunnel: w243 -> [_ _ w247]
          tunnel: [_ _ w245] -> w242
          frame "False", Default {
          }
          frame "root.path" {
            # "Correct root.path"
            n167 = call "Correct_root_path.vi"() -> ()  [unwired: 9 in, 3 out]
          }
          frame "QUIT" {
            n168 = Variant To Data(type=TRUE ("close FP?"), Variant=w247) -> (data=w245:bool)  [unwired: 1 in, 1 out]
            n169 = property on="QUIT" class="Bool (strict)"("Val(Sgnl)"=w245) -> ()  [unwired: 2 in, 2 out]
          }
        }
      }
      event "large histogram": Value Change {
        n170 = event-data() -> ()  [unwired: 1 in, 1 out]
        n171 = Current VI's Path() -> (path=w255:path)
        n172 = Strip Path(path=w255) -> (stripped path=w250:path)  [unwired: 1 out]
        n173 = Strip Path(path=w250) -> (stripped path=w249:path)  [unwired: 1 out]
        n174 = Build Path(base path=w249, name or relative path="image & display") -> (appended path=w253:path)
        n175 = Build Path(base path=w253, name or relative path="large_histogram.vi" ("Variable Name in")) -> (appended path=w251:path)
        n176 = case shown="True" "large histogram" {
          tunnel: w251 -> [w267 w274]
          frame True {
            n177 = Open VI Reference(vi path=w267) -> (vi reference=w260:refnum<vi>, error out=w259:errorcluster)  [unwired: 5 in]
            n178 = invoke class="VI" method="Run VI"(reference=w260, error in=w259, "Wait until done"=FALSE, "Auto Dispose Ref"=TRUE ("Auto Dispose Reference")) -> (reference out=w265:refnum<vi>, error out=w261:errorcluster)  [unwired: 1 in, 3 out]
            n179 = invoke class="VI" method="FP.Open"(reference=w265, error in=w261, "Activate"=TRUE ("Activate?"), "State"=T27."Standard") -> (reference out=w257:refnum<vi>, error out=w258:errorcluster)  [unwired: 1 in, 3 out]
            n180 = Close Reference(reference=w257, error in (no error)=w258) -> ()  [unwired: 1 out]
          }
          frame False {
            n181 = Open VI Reference(vi path=w274) -> (vi reference=w271:refnum<vi>, error out=w270:errorcluster)  [unwired: 5 in]
            n182 = invoke class="VI" method="FP.Close"(reference=w271, error in=w270) -> (reference out=w268:refnum<vi>, error out=w269:errorcluster)  [unwired: 1 in, 1 out]
            n183 = invoke class="VI" method="Abort VI"(reference=w268, error in=w269) -> (reference out=w273:refnum<vi>, error out=w272:errorcluster)  [unwired: 1 in, 1 out]
            n184 = Close Reference(reference=w273, error in (no error)=w272) -> ()  [unwired: 1 out]
          }
        }
      }
      event Menu Selection (User) {
        n185 = event-data() -> ("ItemTag"=w275:string)  [unwired: 1 in]
        n186 = case shown="\"Macro Module\"" w275 {
          selector: w275 -> [_ _ _ _ _ _ w351 w359 _ _ _]
          frame Default {
          }
          frame "Help" {
            n187 = call <vilib>:"Open URL in Default Browser (string).vi"("URL"="http://sciscan.scientifica.uk.com/") -> ()  [unwired: 5 in, 2 out]
          }
          frame "Macro Module" {
            n188 = call "get all running vis.vi"() -> ("RunningVIRefs"=w281:refnum<vi>[])  [unwired: 11 in]
            n189 = for {
              tunnel: w281 -> [w298] mode=indexing
              tunnel: "MacroGUI_MD.vi" ("ItemTag") -> [w294]
              tunnel: [w297] -> w278
              tunnel: [w296] -> w279
              stop <- w297 stop-if-true
              n190 = property class="VI"(reference=w298) -> (reference out=w296:refnum<vi>, "Name"=w295:string)  [unwired: 1 in, 1 out]
              n191 = Equal?(x=w295, y=w294) -> (x = y?=w297:bool)
            }
            n192 = case shown="True" w278 {
              tunnel: w279 -> [_ w289]
              frame False {
                n193 = One Button Dialog(message="Missing Plugin") -> ()  [unwired: 1 in, 1 out]
              }
              frame True {
                n194 = property class="VI"(reference=w289, "FP.State"=T27."Standard" ("Front Panel Window:State")) -> (reference out=w288:refnum<vi>, error out=w287:errorcluster)  [unwired: 1 in]
                n195 = property class="VI"(reference=w288, error in=w287, "FP.Behavior"=T28."Default" ("Front Panel Window:Behavior")) -> (reference out=w284:refnum<vi>, error out=w285:errorcluster)
                n196 = Close Reference(reference=w284, error in (no error)=w285) -> ()  [unwired: 1 out]
                n197 = First Call?() -> (First Call?: T/F=w283:bool)
                n198 = case shown="True" w283 {
                  frame False {
                  }
                  frame True {
                    n199 = call "GFG_core.vi"("Variable Name in"="SciScript_MD_first_launch", "Variant in"=TRUE, "Action"=enum16{"Init", "Set", "Get"}."Set") -> ()  [unwired: 10 in, 7 out]
                  }
                }
              }
            }
          }
          frame "Position Save Module" {
            n200 = call "get all running vis.vi"() -> ("RunningVIRefs"=w302:refnum<vi>[])  [unwired: 11 in]
            n201 = for {
              tunnel: w302 -> [w315] mode=indexing
              tunnel: "PositionSave_coMD.vi" ("ItemTag") -> [w311]
              tunnel: [w314] -> w300
              tunnel: [w313] -> w299
              stop <- w314 stop-if-true
              n202 = property class="VI"(reference=w315) -> (reference out=w313:refnum<vi>, "Name"=w312:string)  [unwired: 1 in, 1 out]
              n203 = Equal?(x=w312, y=w311) -> (x = y?=w314:bool)
            }
            n204 = case shown="True" w300 {
              tunnel: w299 -> [_ w309]
              frame False {
                n205 = One Button Dialog(message="Missing Plugin") -> ()  [unwired: 1 in, 1 out]
              }
              frame True {
                n206 = call "refresh source enum.vi"() -> ()  [unwired: 12 in]
                n207 = property class="VI"(reference=w309, "FP.State"=T27."Standard" ("Front Panel Window:State")) -> (reference out=w308:refnum<vi>, error out=w307:errorcluster)  [unwired: 1 in]
                n208 = property class="VI"(reference=w308, error in=w307, "FP.Behavior"=T28."Default" ("Front Panel Window:Behavior")) -> (reference out=w304:refnum<vi>, error out=w305:errorcluster)
                n209 = Close Reference(reference=w304, error in (no error)=w305) -> ()  [unwired: 1 out]
              }
            }
          }
          frame "OME Module" {
            n210 = call "get all running vis.vi"() -> ("RunningVIRefs"=w319:refnum<vi>[])  [unwired: 11 in]
            n211 = for {
              tunnel: w319 -> [w337] mode=indexing
              tunnel: "OME_coMD.vi" ("ItemTag") -> [w333]
              tunnel: [w336] -> w317
              tunnel: [w335] -> w316
              stop <- w336 stop-if-true
              n212 = property class="VI"(reference=w337) -> (reference out=w335:refnum<vi>, "Name"=w334:string)  [unwired: 1 in, 1 out]
              n213 = Equal?(x=w334, y=w333) -> (x = y?=w336:bool)
            }
            n214 = case shown="True" w317 {
              tunnel: w316 -> [_ w328]
              frame False {
                n215 = One Button Dialog(message="Missing Plugin") -> ()  [unwired: 1 in, 1 out]
              }
              frame True {
                n216 = property class="VI"(reference=w328, "FP.State"=T27."Standard" ("Front Panel Window:State")) -> (reference out=w327:refnum<vi>, error out=w326:errorcluster)  [unwired: 1 in]
                n217 = property class="VI"(reference=w327, error in=w326, "FP.Behavior"=T28."Default" ("Front Panel Window:Behavior")) -> (reference out=w323:refnum<vi>, error out=w324:errorcluster)
                n218 = Close Reference(reference=w323, error in (no error)=w324) -> (error out=w322:errorcluster)
                n219 = First Call?() -> (First Call?: T/F=w321:bool)
                n220 = case shown="True" w321 {
                  tunnel: w322 -> [_ _]
                  frame False {
                  }
                  frame True {
                    n221 = disable-structure shown="Disabled" {
                      frame Disabled {
                        n222 = call "GFG_core.vi"("Variable Name in"="OME_MD_first_launch", "Variant in"=TRUE, "Action"=enum16{"Init", "Set", "Get"}."Set") -> ()  [unwired: 10 in, 7 out]
                      }
                      frame Enabled {
                      }
                    }
                  }
                }
              }
            }
          }
          frame "Uncaging" {
            n223 = call <vilib>:"Application Directory.vi"() -> ("Application Directory"=w344:path)
            n224 = Build Path(base path=w344, name or relative path="Parallel Uncaging Module\\Uncaging UI\\Uncaging Dual.vi") -> (appended path=w346:path)
            n225 = Open VI Reference(vi path=w346) -> (vi reference=w343:refnum<vi>)  [unwired: 5 in, 1 out]
            n226 = invoke class="VI" method="FP.Open"(reference=w343) -> (reference out=w342:refnum<vi>, error out=w341:errorcluster)  [unwired: 4 in, 3 out]
            n227 = invoke class="VI" method="Run VI"(reference=w342, error in=w341, "Wait until done"=FALSE ("Wait Until Done")) -> (reference out=w340:refnum<vi>, error out=w339:errorcluster)  [unwired: 2 in, 3 out]
            n228 = Close Reference(reference=w340, error in (no error)=w339) -> (error out=w338:errorcluster)
            n229 = call <vilib>:"Clear Errors.vi"("error in (no error)"=w338) -> ()  [unwired: 5 in, 2 out]
          }
          frame "Load HW Settings" {
            n230 = call "Settings IO.vi"("SettingsFileIO_Commands"=Settings_IO_Commands."Read HW Settings") -> ("Error Out"=w350:errorcluster, "Cancelled?"=w349:bool, "Settings Array OUT"=w348:T30[])  [unwired: 8 in]
            n231 = case shown="False" w349 {
              tunnel: w351 -> [w355 _]
              tunnel: w350 -> [w354 _]
              tunnel: w348 -> [w353 _]
              frame False {
                n232 = call "Dialog Load Settings.vi"("Error In"=w354, "Title Bar String"=w355, "Settings IN"=w353) -> ()  [unwired: 7 in, 2 out]
              }
              frame True {
              }
            }
          }
          frame "Load Config. Settings" {
            n233 = call "Settings IO.vi"("SettingsFileIO_Commands"=Settings_IO_Commands."Read Config Settings") -> ("Error Out"=w358:errorcluster, "Cancelled?"=w357:bool, "Settings Array OUT"=w356:T30[])  [unwired: 8 in]
            n234 = case shown="False" w357 {
              tunnel: w359 -> [w363 _]
              tunnel: w358 -> [w362 _]
              tunnel: w356 -> [w361 _]
              frame False {
                n235 = call "Dialog Load Settings.vi"("Error In"=w362, "Title Bar String"=w363, "Settings IN"=w361) -> ()  [unwired: 7 in, 2 out]
              }
              frame True {
              }
            }
          }
          frame "Save HW Settings" {
            n236 = call "FGV_Settings IO Rule.vi"("Command_Settings IO Rule"=T14."Get Specified Settings", "Settings Type IN"="HW Settings") -> ("Specified Settings (OUT)"=w365:string[])  [unwired: 7 in, 2 out]
            n237 = for {
              tunnel: w365 -> [w370] mode=indexing
              tunnel: [w369] -> w364 mode=indexing
              n238 = call "GFG_core.vi"("Variable Name in"=w370) -> ("Variant Out"=w371:variant)  [unwired: 12 in, 6 out]
              n239 = Bundle By Name(cluster=T30 {"Variable Name"="", "Value (Variant)"=variant, "data type"=""}, "Variable Name"=w370, "Value (Variant)"=w371) -> (w369:T30)
            }
            n240 = call "Settings IO.vi"("SettingsFileIO_Commands"=Settings_IO_Commands."Write HW Settings", "Settings Array IN"=w364) -> ()  [unwired: 7 in, 3 out]
          }
          frame "Save Config. Settings" {
            n241 = call "FGV_Settings IO Rule.vi"("Command_Settings IO Rule"=T14."Get Specified Settings", "Settings Type IN"="Configuration Settings") -> ("Specified Settings (OUT)"=w374:string[])  [unwired: 7 in, 2 out]
            n242 = for {
              tunnel: w374 -> [w379] mode=indexing
              tunnel: [w378] -> w373 mode=indexing
              n243 = call "GFG_core.vi"("Variable Name in"=w379) -> ("Variant Out"=w380:variant)  [unwired: 12 in, 6 out]
              n244 = Bundle By Name(cluster=T30 {"Variable Name"="", "Value (Variant)"=variant, "data type"=""}, "Variable Name"=w379, "Value (Variant)"=w380) -> (w378:T30)
            }
            n245 = call "Settings IO.vi"("SettingsFileIO_Commands"=Settings_IO_Commands."Write Config Settings", "Settings Array IN"=w373) -> ()  [unwired: 7 in, 3 out]
          }
          frame "QUIT" {
            n246 = call-poly "GFGpolyGet.vi"("Variable Name in"="QUIT") -> ("output cluster"=w384:T31)  [unwired: 9 in, 1 out]
            n247 = Unbundle By Name(w384) -> ("BooleanRef"=w383:refnum<vi>)
            n248 = property class="Bool"(reference=w383, "Val(Sgnl)"=TRUE) -> ()  [unwired: 1 in, 2 out]
          }
        }
      }
      event "Open All\nSettings": Value Change {
        n249 = event-data() -> ()  [unwired: 1 in, 1 out]
        n250 = case shown="True" "Open All\nSettings" {
          frame False {
            n251 = call "slider tabs open.vi"("close(T)/open(F)"=TRUE) -> ()  [unwired: 11 in]
          }
          frame True {
            n252 = call "slider tabs open.vi"("close(T)/open(F)"=FALSE) -> ()  [unwired: 11 in]
          }
        }
      }
      event "QUIT": Value Change {
        w390 = 0.0
        n253 = event-data() -> ()  [unwired: 1 in, 1 out]
        n254 = for {
          N: 4 -> [_]
          tunnel: "ao taskref" ("Variable Name in") -> [w421]
          tunnel: [w416] -> _ mode=indexing
          i -> [w423]
          n255 = Number To Decimal String(number=w423) -> (decimal integer string=w422:string)  [unwired: 1 in]
          n256 = Concatenate Strings(w421, w422) -> (w420:string)
          n257 = call "GFG_core.vi"("Variable Name in"=w420, "Action"=enum16{"Init", "Set", "Get"}."Get") -> ("Variant Out"=w418:variant, "error out"=w419:errorcluster)  [unwired: 11 in, 5 out]
          n258 = Variant To Data(error in=w419, type=refnum<k21> refnum ("task out"), Variant=w418) -> (data=w415:refnum<k21>, error out=w412:errorcluster)
          n259 = call-poly <vilib>:"DAQmx Write.vi"("task/channels in"=w415, "auto start"=TRUE, "data"=0.0, "error in"=w412) -> ("task out"=w413:refnum<k21>, "error out"=w411:errorcluster)  [unwired: 9 in, 1 out]
          n260 = call <vilib>:"DAQmx Clear Task.vi"("task in"=w413, "error in"=w411) -> ("error out"=w416:errorcluster)  [unwired: 13 in]
        }
        n261 = local write "FOCUS"(FALSE ("FOCUS")) -> ()
        n262 = local write "Record"(FALSE ("Record")) -> ()
        n263 = local write "Cancel"(FALSE ("Cancel")) -> ()
        n264 = call "GFG_core.vi"("Variable Name in"="Laser Power", "Variant in"=w390, "Action"=enum16{"Init", "Set", "Get"}."Set") -> ()  [unwired: 10 in, 7 out]
        n265 = local write "Laser Power"(w390) -> ()
        n266 = call "GFG_core.vi"("Variable Name in"="Cancel", "Variant in"=FALSE ("QUIT"), "Action"=enum16{"Init", "Set", "Get"}."Set") -> ()  [unwired: 10 in, 7 out]
        n267 = call "GFG_core.vi"("Variable Name in"="shutter", "Variant in"=FALSE ("QUIT"), "Action"=enum16{"Init", "Set", "Get"}."Set") -> ()  [unwired: 10 in, 7 out]
        n268 = call "getVIname.vi"() -> ("VI name"=w407:string)  [unwired: 19 in]
        n269 = call "GFG_core.vi"("Variable Name in"="FOCUS", "Variant in"=FALSE ("QUIT"), "Action"=enum16{"Init", "Set", "Get"}."Set") -> ()  [unwired: 10 in, 7 out]
        n270 = call "SendShutdownCommand.vi"("Source VI"=w407) -> ()  [unwired: 11 in]
      }
      event "SCIENTIFICA Button": Value Change {
        n271 = event-data() -> ()  [unwired: 1 in, 1 out]
        n272 = call <vilib>:"Open URL in Default Browser (string).vi"("URL"="http://www.scientifica.uk.com/") -> ()  [unwired: 5 in, 2 out]
      }
      event "advanced settings slider tab", "hist/ref slider tab", "PMT slider tab", "laser power slider tab", "XYZ stage settings slider tab": Mouse Enter; "advanced settings slider tab", "hist/ref slider tab", "PMT slider tab", "laser power slider tab", "XYZ stage settings slider tab": Mouse Leave {
        n273 = event-data() -> ("Type"=w430:T26, "CtlRef"=w427:refnum<vi>)  [unwired: 1 in]
        n274 = case shown="1, Default" w431 {
          tunnel: [0 w438] -> w432
          tunnel: w430 -> [_ w435]
          tunnel: w427 -> [_ w437]
          tunnel: [w433 w436] -> w429
          tunnel: w428 -> [w433 _]
          frame 0 {
          }
          frame 1, Default {
            n275 = Bundle("Type"=w435, "CtlRef"=w437) -> (w436:cluster{"Type":T26, "CtlRef":refnum<vi>})  [unwired: 1 in]
            n276 = case shown="\"Mouse Enter\"" w435 {
              tunnel: [0 150] -> w438
              frame "Mouse Leave", Default {
              }
              frame "Mouse Enter" {
              }
            }
          }
        }
      }
      event "clear prot", "timestamp.prot", "protocol.notes": Value Change {
        n277 = event-data() -> ("CtlRef"=w446:refnum<vi>)  [unwired: 1 in]
        n278 = property class="Ctl"(reference=w446) -> ("Label.Text"=w441:string)  [unwired: 1 in, 2 out]
        n279 = case shown="\"timestamp.prot\"" w441 {
          tunnel: "protocol.notes" -> [w455 w460 _]
          tunnel: [w455 w459 ""] -> w445
          frame "Null", Default {
          }
          frame "timestamp.prot" {
            w461 = "frame.count" ("Variable Name in")
            w456 = "\r"
            n280 = call-poly "GFGpolyGet.vi"("Variable Name in"=w461) -> ("Numeric"=w462:dbl)  [unwired: 8 in, 2 out]
            n281 = Number To Decimal String(number=w462) -> (decimal integer string=w458:string)  [unwired: 1 in]
            n282 = Get Date/Time In Seconds() -> (seconds since 1Jan1904=w465:timestamp)
            n283 = Format Date/Time String(time format string (%c)="%Y-%m-%d %H:%M:%S%2u", seconds (now)=w465) -> (date/time string=w463:string)  [unwired: 1 in]
            n284 = Concatenate Strings(w460, "\n##################\n" ("string"), w463, w456, w461, " " ("string"), w458, w456) -> (w459:string)
          }
          frame "clear prot" {
          }
        }
        n285 = flat-sequence {
          tunnel: w445 -> [w452]
          tunnel: [w454] -> w443
          frame #0 {
            n286 = control-ref of="protocol.notes"() -> (w454:refnum<vi>)
            n287 = Wait (ms)(milliseconds to wait=u32 40) -> ()  [unwired: 1 out]
            n288 = call "GFG_core.vi"("Variable Name in"="protocol.notes", "Variant in"=w452, "Action"=enum16{"Init", "Set", "Get", "Clear"}."Set") -> ()  [unwired: 10 in, 7 out]
          }
        }
        n289 = case shown="\"timestamp.prot\"" w441 {
          tunnel: w443 -> [_ w449]
          frame "False", Default {
          }
          frame "timestamp.prot" {
            n290 = call "String Ctl Cursor to End.vi"("String Reference in"=w449) -> ()  [unwired: 10 in, 1 out]
          }
        }
        n291 = case shown="\"timestamp.prot\"" w441 {
          frame Default {
          }
          frame "timestamp.prot" {
            n292 = flat-sequence {
              frame #0 {
                n293 = Wait (ms)(milliseconds to wait=u32 100) -> ()  [unwired: 1 out]
              }
              frame #1 {
              }
            }
          }
          frame "clear prot" {
            n294 = flat-sequence {
              frame #0 {
                n295 = Wait (ms)(milliseconds to wait=u32 100) -> ()  [unwired: 1 out]
              }
              frame #1 {
              }
            }
          }
        }
      }
      event "save prot": Value Change {
        w480 = "\\" ("string")
        n296 = event-data() -> ()  [unwired: 1 in, 1 out]
        n297 = flat-sequence {
          frame #0 {
            n298 = Wait (ms)(milliseconds to wait=u32 100) -> ()  [unwired: 1 out]
          }
          frame #1 {
          }
        }
        n299 = Get Date/Time In Seconds() -> (seconds since 1Jan1904=w470:timestamp)
        n300 = call-poly "GFGpolyGet.vi"("Variable Name in"="root.path") -> ("Path"=w485:path)  [unwired: 8 in, 2 out]
        n301 = Format Date/Time String(time format string (%c)="%Y_%m_%d\\", seconds (now)=w470) -> (date/time string=w481:string)  [unwired: 1 in]
        n302 = Format Date/Time String(time format string (%c)="%Y%m%d_%H_%M_%S", seconds (now)=w470) -> (date/time string=w469:string)  [unwired: 1 in]
        n303 = Path To String(path=w485) -> (string=w482:string)
        n304 = Concatenate Strings(w482, w480, w481, w480, w469, ".notes.txt" ("string")) -> (w475:string)
        n305 = local read "protocol.notes"() -> (w468:string)
        n306 = Search and Replace String(replace all?=TRUE ("replace all? (F)"), input string=w475, search string="[? < > ; ' , * | \" \\t \\r \\n \\s]+", replace string="_" ("replace string (\"\")")) -> (result string=w479:string)  [unwired: 4 in, 3 out]
        n307 = String To Path(string=w479) -> (path=w474:path)
        n308 = call "checkandcreatefoldersforfullpath.vi"("Path IN"=w474) -> ("Path OUT"=w473:path)  [unwired: 4 in]
        n309 = Write to Text File(file (use dialog)=w473, text=w468) -> ()  [unwired: 2 in, 3 out]
      }
    }
  }
  n310 = flat-sequence {
    tunnel: [w492] -> w7
    tunnel: w8 -> [w492]
    frame #0 {
      w491 = dbl[] [4.0, 7.0, 9.0]  # Arbitrary
      w488 = T20."Disabled and Grayed Out" ("Disabled")
      # "Disable arbitrary pixel resolutions, if a standard resolution is selected on start-up."
      n311 = call-poly "GFGpolyGet.vi"("Variable Name in"="pixel.resolution") -> ("Numeric"=w502:dbl)  [unwired: 8 in, 2 out]
      n312 = call-poly "GFGpolyGet.vi"("Variable Name in"="nomin.x.pixels.CtrlRef") -> ("output cluster"=w495:T31)  [unwired: 9 in, 1 out]
      n313 = call-poly "GFGpolyGet.vi"("Variable Name in"="y.pixels.CtrlRef") -> ("output cluster"=w497:T31)  [unwired: 9 in, 1 out]
      n314 = Equal?(x=w491, y=w502) -> (x = y?=w490:bool[])
      n315 = Or Array Elements(Boolean array=w490) -> (logical OR=w489:bool)
      n316 = Unbundle By Name(w495) -> ("DigitalRef"=w494:refnum<vi>)
      n317 = Unbundle By Name(w497) -> ("DigitalRef"=w498:refnum<vi>)
      n318 = Select(t=T20."Enabled" ("Disabled"), s=w489, f=w488) -> (s? t:f=w493:T20)
      n319 = property class="DigNum"(reference=w494, "DisabledEnum"=w488) -> ()  [unwired: 1 in, 2 out]
      n320 = property class="DigNum"(reference=w498, "DisabledEnum"=w493) -> ()  [unwired: 1 in, 2 out]
    }
  }
  n321 = flat-sequence {
    tunnel: [w505] -> w14
    tunnel: [w504] -> w13
    tunnel: w7 -> [w503]
    tunnel: [w503] -> w12
    tunnel: [w503] -> _
    frame #0 {
      n322 = call-poly "GFGpolyGet.vi"("Variable Name in"="version") -> ("Found/Replaced"=w504:bool, "String"=w505:string)  [unwired: 9 in]
    }
  }
  n323 = case "Add software version in title bar, if found" shown="True" w13 {
    tunnel: w12 -> [w507 w510]
    tunnel: w14 -> [_ w509]
    tunnel: [w507 w508] -> w6
    frame False {
    }
    frame True {
      n324 = control-ref of="This VI"() -> (w518:refnum<vi>)
      n325 = property class="VI"(reference=w518, error in=w510) -> (reference out=w514:refnum<vi>, error out=w513:errorcluster, "Front Panel.Title"=w517:string)
      n326 = Concatenate Strings(w517, " " ("string"), w509) -> (w515:string)
      n327 = property class="VI"(reference=w514, error in=w513, "Front Panel.Title"=w515) -> (reference out=w512:refnum<vi>, error out=w511:errorcluster)
      n328 = Close Reference(reference=w512, error in (no error)=w511) -> (error out=w508:errorcluster)
    }
  }
  n329 = flat-sequence {
    tunnel: w37 -> [w523]
    tunnel: [w523] -> w29
    tunnel: w4 -> [_]
    tunnel: [w525] -> w19
    tunnel: w29 -> [w525]
    tunnel: w19 -> [w528]
    tunnel: [w528] -> w18
    tunnel: w17 -> [w527]
    tunnel: [w526] -> w10
    tunnel: w18 -> [w537]
    tunnel: w10 -> [w536]
    tunnel: [w536] -> w9
    tunnel: w9 -> [w541]
    frame #0 {
      # "Reset laser power"
      n330 = local write "piezo.active"(FALSE ("close FP?")) -> ()
      n331 = call "GFG_core.vi"("Variable Name in"="Laser.Power" ("Variable Name"), "Variant in"=0.0, "Action"=enum16{"Init", "Set", "Get", "Clear"}."Set") -> ()  [unwired: 10 in, 7 out]
    }
    frame #1 {
      n332 = call "close modules.vi"("close FP?"=TRUE) -> ()  [unwired: 11 in]
    }
    frame #2 {
      n333 = Empty Array?(array=w527) -> (empty?=w526:bool)
      n334 = case "Write relative positions to inactive HS INIs" shown="False" w526 {
        tunnel: w527 -> [w535 _]
        tunnel: [w531 _] -> _
        tunnel: [w530 _] -> _
        frame False {
          w529 = "stage.control" ("Variable Name")
          w532 = string[] ["Xoffset", "Yoffset", "Zoffset"] ("Variables Names In")
          n335 = Index Array(array=w535) -> (element #1=w534:path, element #2=w533:path)  [unwired: 2 in]
          n336 = call "ReadSubsetofGFGandWritetoINI.vi"("Key Section (_)"=w529, "Variable Names In"=w532, "Path"=w534) -> ("error out"=w531:errorcluster)  [unwired: 8 in]
          n337 = call "ReadSubsetofGFGandWritetoINI.vi"("Key Section (_)"=w529, "Variable Names In"=w532, "Path"=w533) -> ("error out"=w530:errorcluster)  [unwired: 8 in]
        }
        frame True {
          # "Standalone version. No further action required."
        }
      }
    }
    frame #3 {
      n338 = Not(x=w537) -> (.not. x?=w538:bool)
      n339 = call "ReadGFGandWriteToINI.vi"() -> ("error out"=w539:errorcluster)  [unwired: 11 in]
      n340 = local write "QUIT"(w538) -> ()
      n341 = call "GFG_core.vi"("error in (no error)"=w539, "Action"=enum16{"Init", "Set", "Get"}."Init") -> ()  [unwired: 11 in, 7 out]
    }
    frame #4 {
      n342 = case shown="True" w541 {
        frame False {
          # "If this is not a standalone version, all DAQ devices will be reset when quitting the MAIN VI only. Don't do it here!"
        }
        frame True {
          # "If this is the standalone version, reset all DAQ devices."
          n343 = flat-sequence "Wait until SciScan stopped\nand reset all DAQ devices" {
            frame #0 {
              n344 = Wait (ms)(milliseconds to wait=u32 200) -> ()  [unwired: 1 out]
            }
            frame #1 {
              n345 = call "Reset_DAQ.vi"() -> ()  [unwired: 11 in, 1 out]
            }
          }
        }
      }
    }
  }
  n346 = flat-sequence {
    tunnel: w6 -> [w543]
    tunnel: [w543] -> w4
    frame #0 {
      # "You may start \nclicking now..."
      n347 = call <vilib>:"Unset Busy.vi"() -> ()  [unwired: 11 in, 1 out]
    }
  }
  n348 = flat-sequence "Monitor if the Main UI crashed - If so, make QUIT button visible." {
    tunnel: w4 -> [_]
    frame #0 {
      n349 = call "getCallerVIname.vi"() -> ("VI name"=w545:string)  [unwired: 19 in]
      n350 = Empty String/Path?(string/path=w545) -> (empty?=w544:bool)
      n351 = case shown="False" w544 {
        frame True {
          # "There is no MAIN UI. Do nothing."
        }
        frame False {
          n352 = while {
            stop <- w546 stop-if-true
            n353 = event shown="[1] \"QUIT\": Value Change" {
              selector: _ -> [_ _]
              dyn-events: _ -> [_ _]
              timeout: _ -> [_ _]
              tunnel: [_ w550] -> w546
              event "MAIN UI responsive? (F)": Value Change {
                n354 = event-data() -> ()  [unwired: 1 in, 1 out]
                n355 = Not(x="MAIN UI responsive? (F)") -> (.not. x?=w548:bool)
                n356 = property on="QUIT" class="Bool (strict)"("Visible"=w548) -> ()  [unwired: 2 in, 2 out]
              }
              event "QUIT": Value Change {
                w550 = TRUE  # QUIT
                n357 = event-data() -> ()  [unwired: 1 in, 1 out]
                n358 = property on="MAIN UI responsive? (F)" class="Bool (strict)"() -> ("Value"=w549:bool)  [unwired: 2 in, 2 out]
                n359 = case "If not responsive, QUIT all other VIs (including MAIN UI)." shown="False" w549 {
                  frame False {
                    n360 = control-ref of="This Application"() -> (w552:refnum<vi>)
                    n361 = property class="App"(reference=w552) -> (reference out=w554:refnum<vi>, error out=w555:errorcluster, "App.AllVIs"=w553:string[])  [unwired: 1 in]
                    n362 = Close Reference(reference=w554, error in (no error)=w555) -> (error out=w551:errorcluster)
                    n363 = for {
                      tunnel: w553 -> [w562] mode=indexing
                      tunnel: w551 -> [w557]
                      n364 = Open VI Reference(vi path=w562, error in (no error)=w557) -> (vi reference=w561:refnum<vi>, error out=w560:errorcluster)  [unwired: 4 in]
                      n365 = invoke class="VI" method="Abort VI"(reference=w561, error in=w560) -> (reference out=w559:refnum<vi>, error out=w558:errorcluster)  [unwired: 1 in, 1 out]
                      n366 = Close Reference(reference=w559, error in (no error)=w558) -> (error out=w556:errorcluster)
                      n367 = call <vilib>:"Clear Errors.vi"("error in (no error)"=w556) -> ()  [unwired: 5 in, 2 out]
                    }
                  }
                  frame True {
                    # "MAIN UI still responsive. Keep it running!"
                  }
                }
              }
            }
          }
        }
      }
    }
  }
